vi "BML_Reg_Scan.vi"() -> ()   [LabVIEW 2016]
panel:
  out "Array 2":string[](array[string])
  out "Array":u16[](array[numeric]) format="%x"
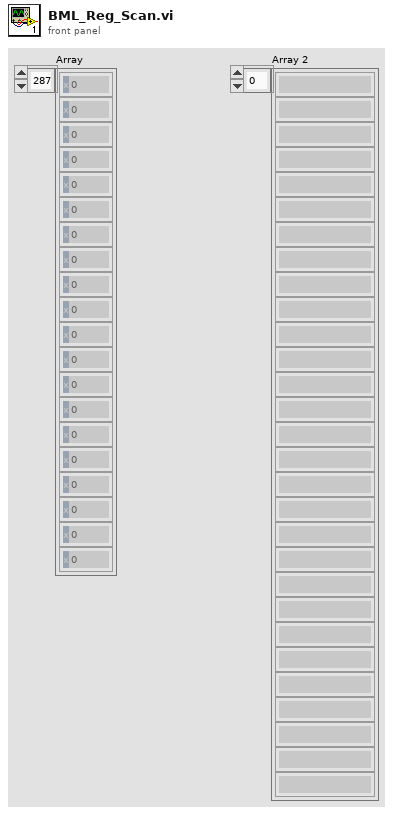
[diagram p1: front panel]
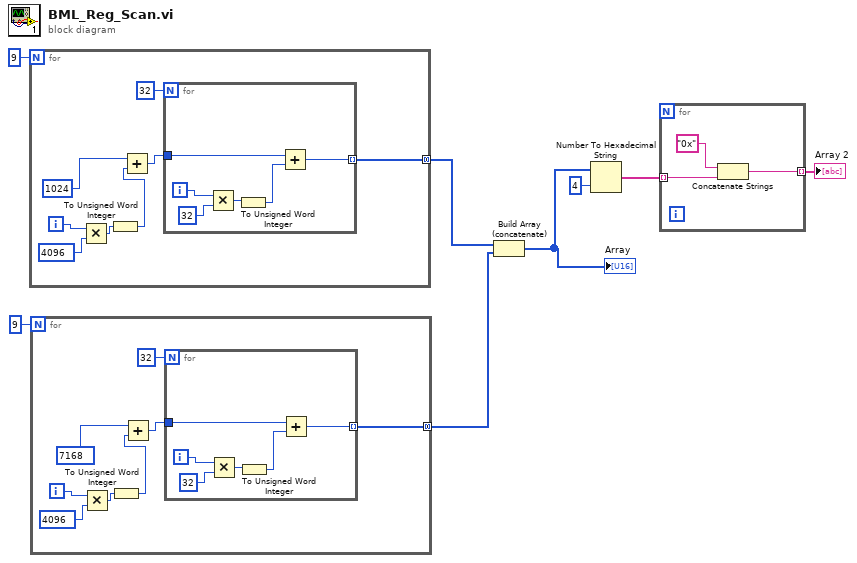
[diagram p0: block diagram]
diagram:
  n1 = for {
    N: 9 -> [_]
    tunnel: [w9] -> w6 mode=concatenating
    i -> [w15]
    n2 = Multiply(x=w15, y=4096) -> (x*y=w12:i32)
    n3 = To Unsigned Word Integer(number=w12) -> (unsigned 16bit integer=w11:u16)
    n4 = Add(x=u16 1024, y=w11) -> (x+y=w10:u16)
    n5 = for {
      N: 32 -> [_]
      tunnel: w10 -> [w20]
      tunnel: [w17] -> w9 mode=indexing
      i -> [w21]
      n6 = Multiply(x=w21, y=32) -> (x*y=w19:i32)
      n7 = To Unsigned Word Integer(number=w19) -> (unsigned 16bit integer=w18:u16)
      n8 = Add(x=w20, y=w18) -> (x+y=w17:u16)
    }
  }
  n9 = for {
    N: 9 -> [_]
    tunnel: [w23] -> w5 mode=concatenating
    i -> [w29]
    n10 = Multiply(x=w29, y=4096) -> (x*y=w26:i32)
    n11 = To Unsigned Word Integer(number=w26) -> (unsigned 16bit integer=w25:u16)
    n12 = Add(x=u16 7168, y=w25) -> (x+y=w24:u16)
    n13 = for {
      N: 32 -> [_]
      tunnel: w24 -> [w34]
      tunnel: [w31] -> w23 mode=indexing
      i -> [w35]
      n14 = Multiply(x=w35, y=32) -> (x*y=w33:i32)
      n15 = To Unsigned Word Integer(number=w33) -> (unsigned 16bit integer=w32:u16)
      n16 = Add(x=w34, y=w32) -> (x+y=w31:u16)
    }
  }
  n17 = Build Array (concatenate)(w6, w5) -> (w4:u16[])
  "Array" <- w4
  n18 = Number To Hexadecimal String(1:i16 4 ("width (-)"), 2:w4) -> (0:w2:string[])
  n19 = for {
    tunnel: w2 -> [w38] mode=indexing
    tunnel: [w37] -> w1 mode=indexing
    n20 = Concatenate Strings("0x" ("string"), w38) -> (w37:string)
  }
  "Array 2" <- w1
